vi "hashFunctionConstructor.vi"(11 "Hash Function":refnum<vi>) -> (0 "error out":errorcluster, 3 "HashMap out":refnum<class "HashMap.lvclass">)   [LabVIEW 2017, in "HashMap.lvclass"]
uses:
  <userlib>/836-Library/Data_Structures/HashMap/HashMap.lvclass
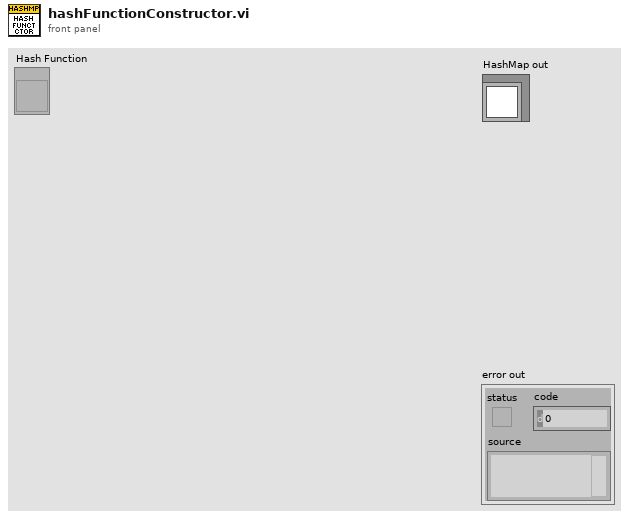
[diagram p1: front panel]
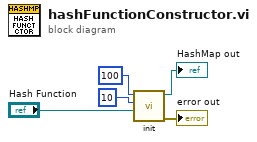
[diagram p0: block diagram]
diagram:
  n1 = call <userlib>:"init.vi"("Hash Function"="Hash Function", "Bucket Size"=u32 10, "NumBuckets"=100) -> ("error out"=→"error out":errorcluster, "HashMap out"=→"HashMap out":refnum<class "HashMap.lvclass">)  [unwired: 7 in]
